vi "Configure Calibration Output.vi"(8 "error in (no error)":errorcluster, 10 "Calibration Output Type (0: Trigger)":i32(ring) items=["Trigger", "Mask", "Waveform Generator"], 11 "VISA resource name":refnum<visa-resource-name>) -> (0 "error out":errorcluster, 3 "VISA resource name out":refnum<visa-resource-name>)   [LabVIEW 2010, in "Agilent 2000 3000 X-Series.lvlib"]
doc: "Sets the signal that is available on the rear panel TRIG OUT BNC."
uses:
  <instrlib>/Agilent 2000 3000 X-Series/Agilent 2000 3000 X-Series.lvlib
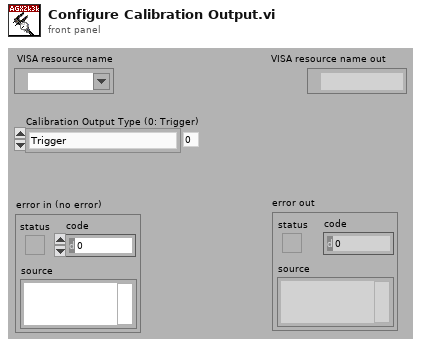
[diagram p1: front panel]
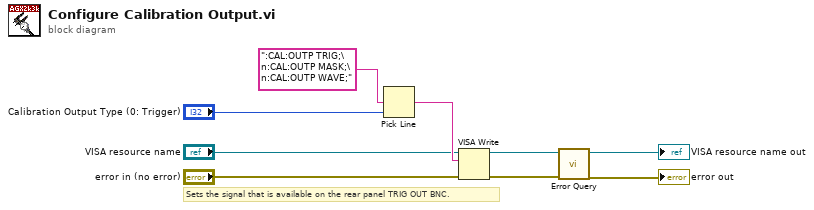
[diagram p0: block diagram]
diagram:
  # "Sets the signal that is available on the rear panel TRIG OUT BNC."
  n1 = Pick Line(multi-line string=":CAL:OUTP TRIG;\n:CAL:OUTP MASK;\n:CAL:OUTP WAVE;", line index="Calibration Output Type (0: Trigger)") -> (output string=w7:string)  [unwired: 1 out]
  n2 = VISA Write(VISA resource name="VISA resource name", write buffer=w7, error in (no error)="error in (no error)") -> (VISA resource name out=w4:refnum<visa-resource-name>, error out=w3:errorcluster)  [unwired: 1 out]
  n3 = call <instrlib>:"Error Query.vi"("error in (no error)"=w3, "VISA resource name"=w4) -> ("error out"=→"error out":errorcluster, "VISA resource name out"=→"VISA resource name out":refnum<visa-resource-name>)  [unwired: 8 out]
